vi "load_siglent_csv_file.vi"(6 "filename_in":string, 7 "button_load_csv":bool, 8 "data_available_in":T1, 9 "freq_available in":bool, 10 "s11_data_array_in":dbl[][](array[numeric]), 11 "freq_array_in":dbl[](array[numeric])) -> (0 "data_available_out":T1, 1 "freq_available_out":bool, 2 "s11_data_array_out":dbl[][](array[numeric]), 3 "freq_array_out":dbl[](array[numeric]), 4 "filename_out":string)   [LabVIEW 2025]
panel:
  out "Loaded *.csv-File":string
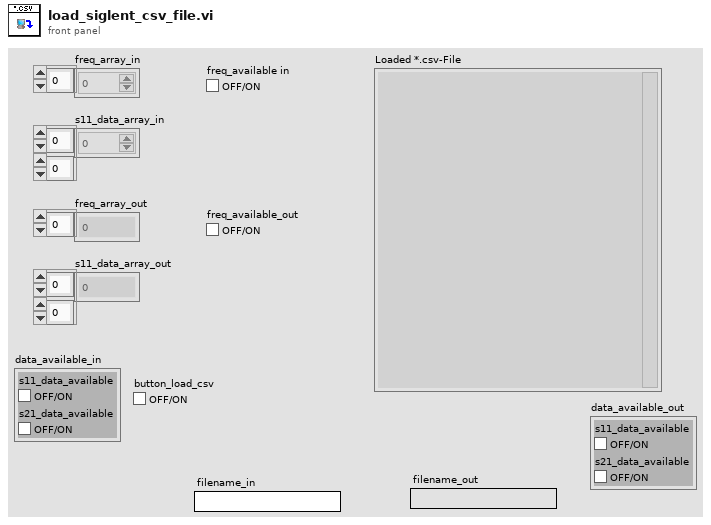
[diagram p1: front panel]
types:
  T1 = cluster{"s11_data_available":bool, "s21_data_available":bool}
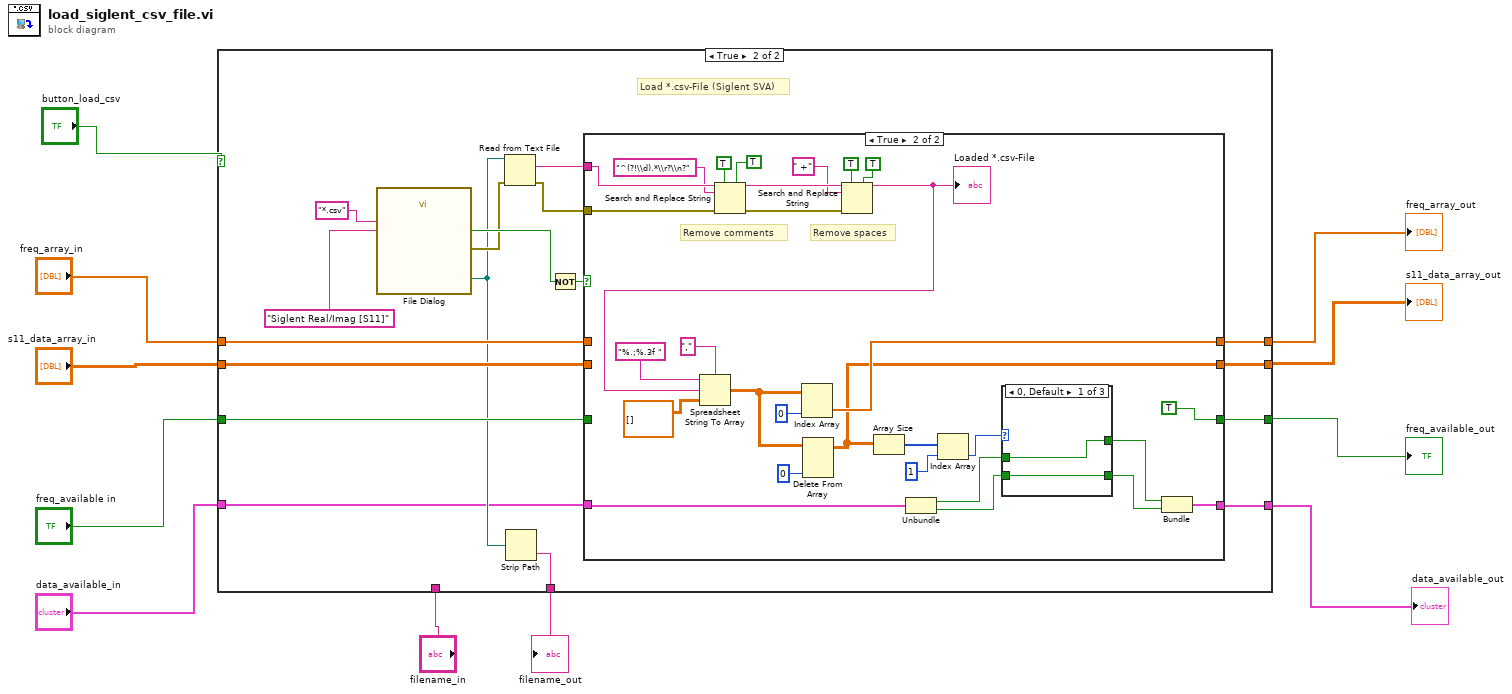
[diagram p0: block diagram]
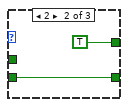
[diagram p4: hidden frame]
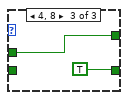
[diagram p5: hidden frame]
diagram:
  n1 = case shown="True" "button_load_csv" {
    tunnel: [w16 w33] -> w8
    tunnel: "freq_array_in" -> [w16 w21]
    tunnel: [w15 w32] -> w7
    tunnel: "s11_data_array_in" -> [w15 w22]
    tunnel: [w14 w31] -> w5
    tunnel: "freq_available in" -> [w14 w23]
    tunnel: [w13 w19] -> w4
    tunnel: "filename_in" -> [w13 _]
    tunnel: "data_available_in" -> [w12 w17]
    tunnel: [w12 w18] -> w1
    frame False {
    }
    frame True {
      # "Load *.csv-File (Siglent SVA)"
      n2 = call "File Dialog"("pattern (all files)"="*.csv" ("pattern label"), "pattern label"="Siglent Real/Imag [S11]") -> ("selected path"=w20:path, "cancelled"=w28:bool, "error out"=w26:errorcluster)  [unwired: 10 in, 1 out]
      n3 = Read from Text File(file (use dialog)=w20, error in=w26) -> (text=w30:string, error out=w27:errorcluster)  [unwired: 2 in, 2 out]
      n4 = Strip Path(path=w20) -> (name=w19:string)  [unwired: 1 out]
      n5 = Not(x=w28) -> (.not. x?=w29:bool)
      n6 = case shown="True" w29 {
        tunnel: [w35 w64] -> w33
        tunnel: [w36 w47] -> w32
        tunnel: [w37 TRUE ("freq_available")] -> w31
        tunnel: w30 -> [_ w59]
        tunnel: w27 -> [_ w58]
        tunnel: w23 -> [w37 _]
        tunnel: w22 -> [w36 _]
        tunnel: w21 -> [w35 _]
        tunnel: [w34 w43] -> w18
        tunnel: w17 -> [w34 w42]
        frame False {
        }
        frame True {
          # "Remove comments"
          # "Remove spaces"
          n7 = Search and Replace String(replace all?=TRUE ("replace all? (F)"), multiline?=TRUE ("multiline? (F)"), input string=w59, search string="^(?!\\d).*\\r?\\n?", error in=w58) -> (result string=w53:string, error out=w52:errorcluster)  [unwired: 3 in, 2 out]
          n8 = Search and Replace String(replace all?=TRUE ("replace all? (F)"), multiline?=TRUE ("replace all? (F)"), input string=w53, search string=" +", error in=w52) -> (result string=w48:string)  [unwired: 3 in, 3 out]
          "Loaded *.csv-File" <- w48
          n9 = Spreadsheet String To Array(delimiter (Tab)="," ("element"), format string="%.;%.3f ", spreadsheet string=w48, array type (2D Dbl)=dbl[][] []) -> (array=w55:dbl[][])
          n10 = Index Array(array=w55, index (col)=0) -> (element=w64:dbl[])  [unwired: 1 in]
          n11 = Delete From Array(array=w55, index (col)=0) -> (array with subset deleted=w47:dbl[][])  [unwired: 2 in, 1 out]
          n12 = Array Size(array=w47) -> (size(s)=w46:i32[])
          n13 = Unbundle(w42) -> ("s11_data_available"=w38:bool, "s21_data_available"=w40:bool)
          n14 = Index Array(array=w46, index=1) -> (element=w44:i32)
          n15 = case shown="0, Default" w44 {
            tunnel: [w67 w70 TRUE] -> w41
            tunnel: w40 -> [w67 w70 _]
            tunnel: [w68 TRUE w72] -> w39
            tunnel: w38 -> [w68 _ w72]
            frame 0, Default {
            }
            frame 2 {
            }
            frame 4, 8 {
            }
          }
          n16 = Bundle("s11_data_available"=w39, "s21_data_available"=w41) -> (w43:T1)  [unwired: 1 in]
        }
      }
    }
  }
  "freq_array_out" <- w8
  "s11_data_array_out" <- w7
  "freq_available_out" <- w5
  "filename_out" <- w4
  "data_available_out" <- w1
